vi "KEN_Query.vi"(0 "System no.":i32=1 min=1 max=4 step=1, 2 "Names to query":string[](array[string]), 5 "error in":errorcluster) -> (14 "Types":string[](array[string]), 19 "error out":errorcluster)   [LabVIEW 2020]
doc: "Returns active coordinate systems. The returned information depends on the arguments used. If no argument is set, all active coordinate systems are returned. The KEN? command sets an error code if a coordinate system with the specified name is not defined.\n\nC-887, F-206, M-8X0: Only for GCS syntax version = GCS 2.0 or higher (Check with CSV?.vi. If CSV?.vi is not supported, syntax version is GCS 1.0)."
panel:
  # "Returns enabled coordinate systems. The returned information depends \non the arguments used."
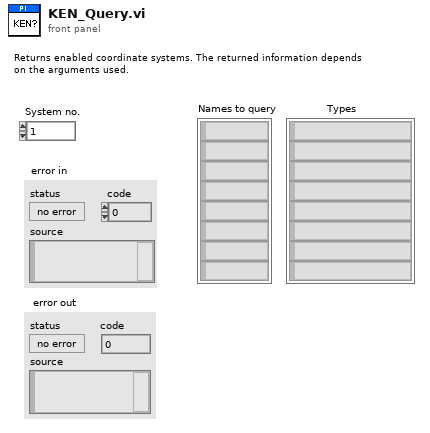
[diagram p1: front panel]
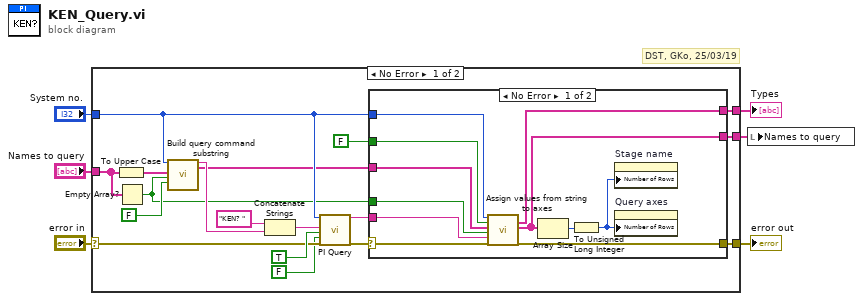
[diagram p0: block diagram]
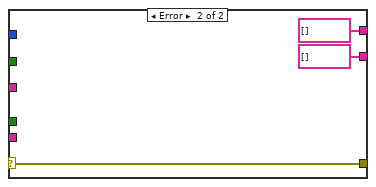
[diagram p2: hidden frame]
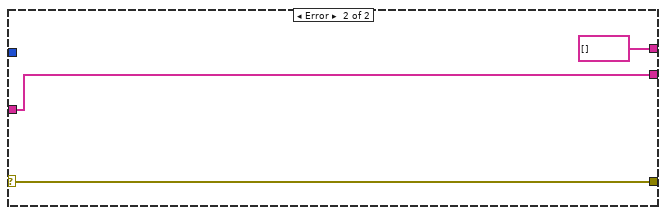
[diagram p3: hidden frame]
diagram:
  # "DST, GKo, 25/03/19"
  n1 = case shown="No Error" "error in" {
    selector: "error in" -> [w13 w40]
    tunnel: "Names to query" -> [w9 w39]
    tunnel: [w15 w40] -> w5
    tunnel: "System no." -> [w19 _]
    tunnel: [w17 string[] [] ("Strings")] -> w3
    tunnel: [w7 w39] -> w1
    frame No Error {
      n2 = To Upper Case(1:w9) -> (0:w21:string[])
      n3 = Empty Array?(array=w9) -> (empty?=w8:bool)
      n4 = call "Build query command substring.vi"("System no."=w19, "Axes to query in"=w21, "Query\nAll axes?"=w8, "For all axes: use\nAxis identifier?"=FALSE ("For all axes: use\nAxis identifier?")) -> ("Command substring"=w20:string, "Axes to query out"=w18:string[])  [unwired: 2 in, 12 out]
      n5 = Concatenate Strings("KEN? ", w20) -> (w22:string)
      n6 = call "PI Query.vi"("System no."=w19, "String to send"=w22, "Attach termination char.?"=TRUE ("Attach Linefeed?"), "Strip spaces?"=FALSE, "error in"=w13) -> ("String read"=w11:string, "error out"=w10:errorcluster)  [unwired: 2 in, 11 out]
      n7 = case shown="No Error" w10 {
        selector: w10 -> [w26 w38]
        tunnel: w19 -> [w35 _]
        tunnel: w18 -> [w34 _]
        tunnel: [w33 string[] [] ("Strings")] -> w17
        tunnel: [w32 w38] -> w15
        tunnel: FALSE ("Axes related?") -> [w31 _]
        tunnel: w8 -> [w29 _]
        tunnel: w11 -> [w28 _]
        tunnel: [w25 string[] [] ("Queried axes out")] -> w7
        frame No Error {
          n8 = call "Assign values from string to axes.vi"("System no."=w35, "Queried axes"=w34, "All axes queried?"=w29, "Input String"=w28, "error in"=w26, "Axes related?"=w31) -> ("Strings"=w33:string[], "Queried axes out"=w25:string[], "error out"=w32:errorcluster)  [unwired: 3 in, 8 out]
          n9 = Array Size(array=w25) -> (size(s)=w30:i32)
          n10 = To Unsigned Long Integer(number=w30) -> (unsigned 32bit integer=w27:u32)
          n11 = property on="Stage name" class="Arr (strict)"("Number of Rows"=w27) -> ()  [unwired: 2 in, 2 out]
          n12 = property on="Query axes" class="Arr (strict)"("Number of Rows"=w27) -> ()  [unwired: 2 in, 2 out]
        }
        frame Error {
        }
      }
    }
    frame Error {
    }
  }
  "error out" <- w5
  "Types" <- w3
  n13 = local write "Names to query"(w1) -> ()
